vi "setUp.vi"(8 "error in (no error)":errorcluster, 11 "reference in":refnum<class "TestSQliteDatabaseConfiguration.lvclass">) -> (0 "error out":errorcluster, 3 "reference out":refnum<class "TestSQliteDatabaseConfiguration.lvclass">)   [LabVIEW 2020, in "SQlite tests.lvlib" / "TestSQliteDatabaseConfiguration.lvclass"]
doc: "setUp runs prior to the test method during test execution. Use this method to initialize any object data required by your tests."
uses:
  TestSQliteDatabaseConfiguration.lvclass
  <vilib>/addons/_JKI Toolkits/VI Tester/TestCase.llb/TestCase.lvclass
  <vilib>/Utility/sysdir.llb/System Directory Type.ctl
  externals/database-interface/Source/sqlite3/Source/sqlite3.lvclass
  C:/Users/Fred.Guo/Desktop/Database-configuration/externals/database-interface/Source/IDatabase/IDatabase/IDatabase.lvclass
  C:/Users/Fred.Guo/Desktop/Database-configuration/externals/database-interface/Source/sqlite3/Source/sqlite3.lvclass
  C:/Program Files/National Instruments/LabVIEW 2020/vi.lib/addons/_JKI Toolkits/VI Tester/TestCase.llb/TestCase.lvclass
  C:/Users/Fred.Guo/Desktop/Database-configuration/_Test/sqlite configuration database/TestSQliteDatabaseConfiguration.lvclass
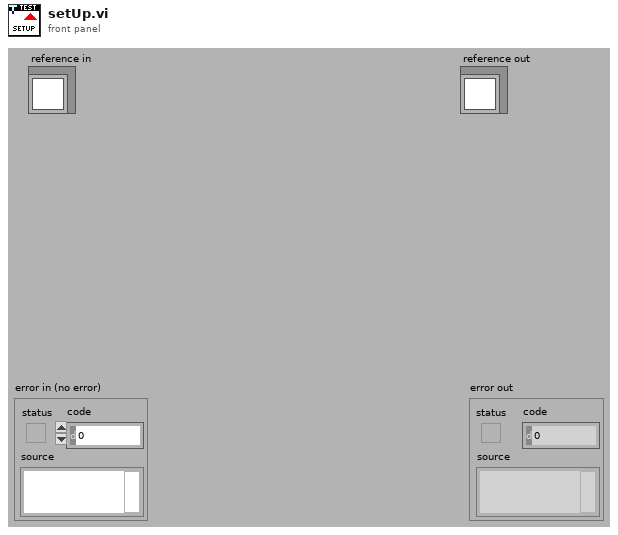
[diagram p1: front panel]
types:
  T1 = typedef "System Directory Type.ctl" = i32
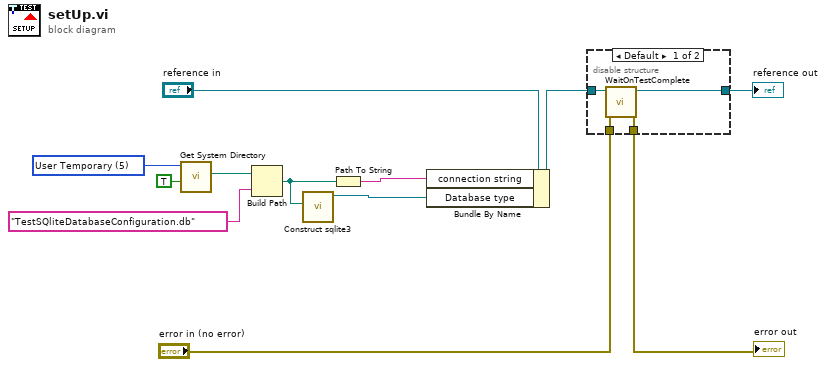
[diagram p0: block diagram]
diagram:
  w7 = T1 5 items=["User Home"=0, "User Desktop"=1, "User Documents"=2, "User Application Data"=3, "User Preferences"=4, "User Temporary"=5, "Public Documents"=6, "Public Application Data"=7, "Public Preferences"=8, "Public Cache"=13, "System Core Libraries"=9, "System Installed Libraries"=10, "Application Files"=11, "Boot Volume Root"=12] ("system directory type")
  n1 = call <vilib>:"Get System Directory.vi"("create directory if not found? (F)"=TRUE, "system directory type"=w7) -> ("system directory"=w5:path)  [unwired: 9 in]
  n2 = Build Path(base path=w5, name or relative path="TestSQliteDatabaseConfiguration.db") -> (appended path=w1:path)
  n3 = call "Construct sqlite3.vi"("DatabaseFilePath"=w1) -> ("sqlite3 out"=w2:refnum<class "sqlite3.lvclass">)  [unwired: 9 in, 1 out]
  n4 = Path To String(path=w1) -> (string=w3:string)
  n5 = Bundle By Name(cluster="reference in", "connection string"=w3, "Database type"=w2) -> (w8:refnum<class "TestSQliteDatabaseConfiguration.lvclass">)
  n6 = disable-structure shown="Default" {
    disable-tunnel: "error in (no error)" -> [w16 w17]
    disable-tunnel: [w15 w17] -> w11
    disable-tunnel: [w14 w18] -> w9
    disable-tunnel: w8 -> [w13 w18]
    frame condition #0 (active) {
      n7 = call <vilib>:"WaitOnTestComplete.vi"("error in (no error)"=w16, "TestCase in"=w13) -> ("error out"=w15:errorcluster, "TestCase out"=w14:refnum<class "TestSQliteDatabaseConfiguration.lvclass">)  [unwired: 8 in]
    }
    frame condition #1 {
    }
  }
  "error out" <- w11
  "reference out" <- w9
